vi "调用对话框.vi"() -> ()   [LabVIEW 2018]
panel:
  out "数值 4":dbl
  out "数值 3":dbl
  in  "停止":bool
  in  "设置":bool
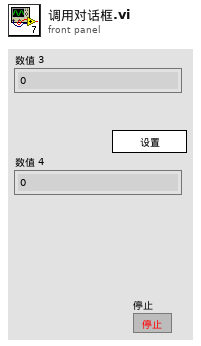
[diagram p1: front panel]
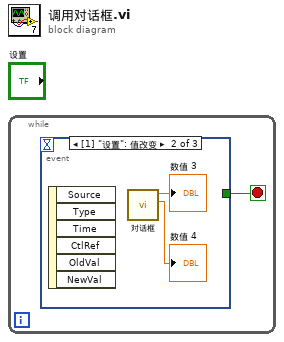
[diagram p0: block diagram]
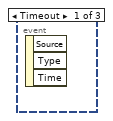
[diagram p2: hidden frame]
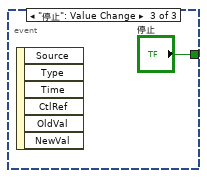
[diagram p3: hidden frame]
diagram:
  n1 = while {
    stop <- w1 stop-if-true
    n2 = event shown="[1] \"设置\": 值改变" {
      selector: _ -> [_ _ _]
      dyn-events: _ -> [_ _ _]
      timeout: _ -> [_ _ _]
      tunnel: [_ _ "停止"] -> w1
      event Timeout {
        n3 = event-data() -> ()  [unwired: 1 in, 3 out]
      }
      event "设置": Value Change {
        n4 = event-data() -> ()  [unwired: 1 in, 6 out]
        n5 = call "对话框.vi"() -> ("数值 4"=→"数值 4":dbl, "数值 3"=→"数值 3":dbl)  [unwired: 10 in]
      }
      event "停止": Value Change {
        n6 = event-data() -> ()  [unwired: 1 in, 6 out]
      }
    }
  }
